vi "五子棋.vi"() -> ()   [LabVIEW 2018]
panel:
  in  "开始游戏":bool
  in  "对弈模式":enum16{"人机对弈", "双人对弈"}(ring)
  in  "重新开始":bool
  in  "退出程序":bool
  out "消息显示":string(combo)
  in  "控制数组":bool[][](array[boolean])
  out "显示数组":bool[][](array[boolean])
  out "当前棋盘状态":u16[][](array[ring])
  # "五  子  棋"
  # "0"
  # "1"
  # "2"
  # "3"
  # "4"
  # "5"
  # "6"
  # "7"
  # "8"
  # "9"
  # "10"
  # "11"
  # "12"
  # "13"
  # "14"
  # "0"
  # "1"
  # "2"
  # "3"
  # "4"
  # "5"
  # "6"
  # "7"
  # "8"
  # "9"
  # "10"
  # "11"
  # "12"
  # "13"
  # "14"
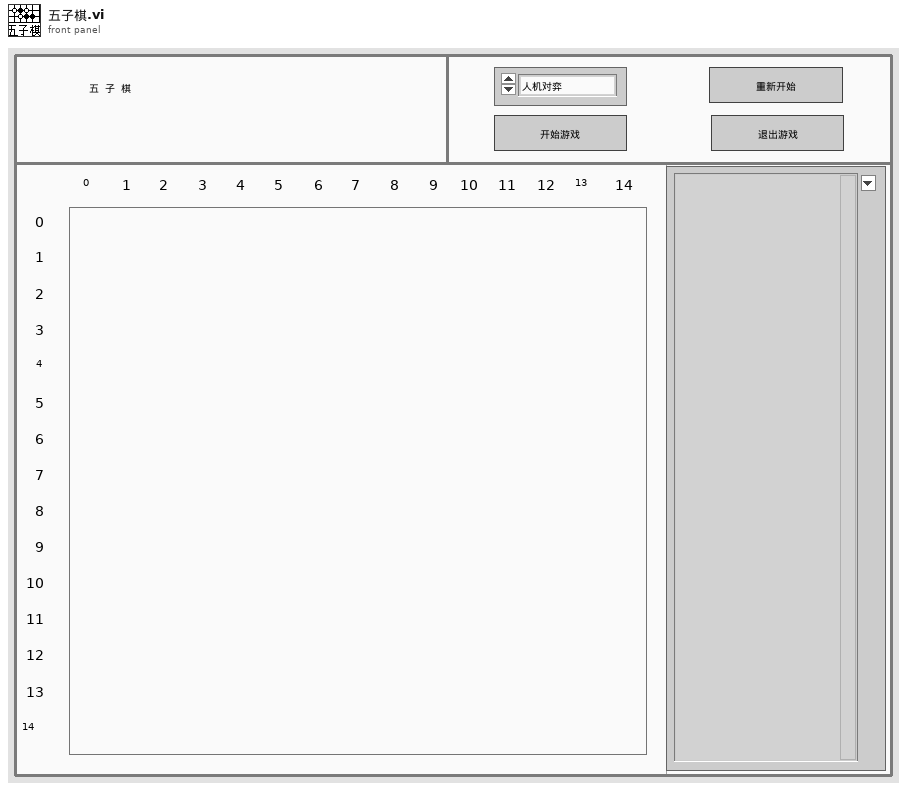
[diagram p1: front panel]
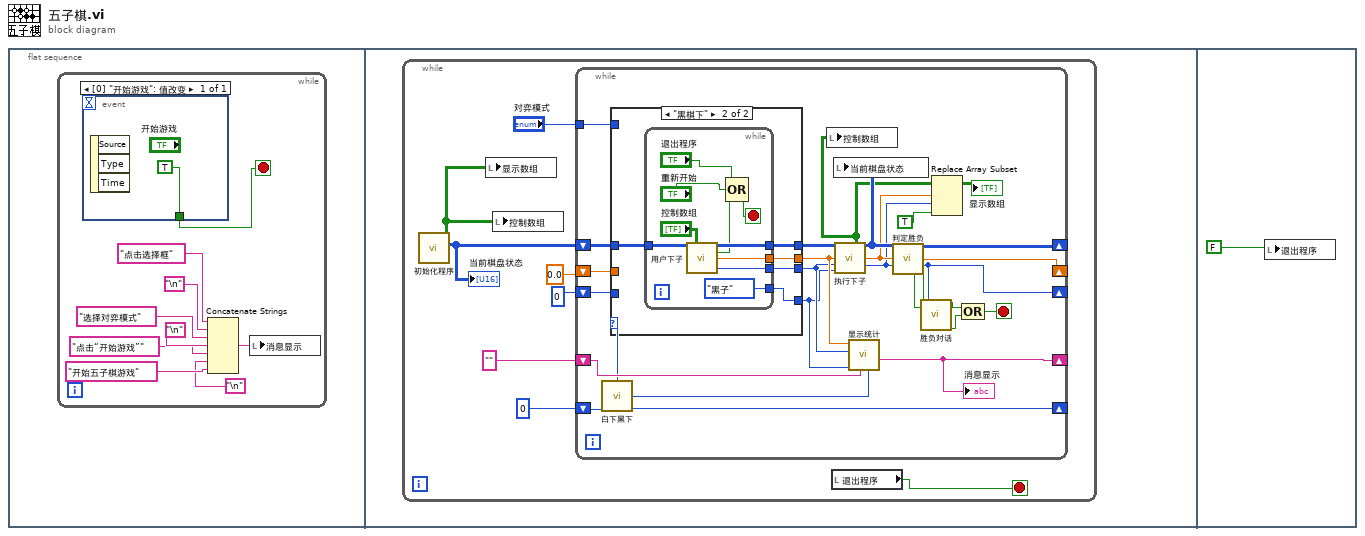
[diagram p0: block diagram]
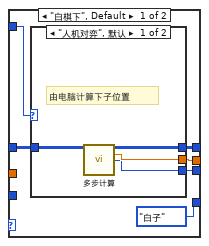
[diagram p2: hidden frame]
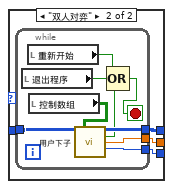
[diagram p3: hidden frame]
diagram:
  n1 = flat-sequence {
    frame #0 {
      n2 = while {
        stop <- w9 stop-if-true
        n3 = event shown="[0] \"开始游戏\": 值改变" {
          selector: _ -> [_]
          dyn-events: _ -> [_]
          timeout: _ -> [_]
          tunnel: [TRUE] -> w9
          event "开始游戏": Value Change {
            n4 = event-data() -> ()  [unwired: 1 in, 3 out]
          }
        }
        n5 = Concatenate Strings("点击选择框", "\n", "选择对弈模式", "\n", "点击“开始游戏”", "\n", "开始五子棋游戏") -> (w5:string)
        n6 = local write "消息显示"(w5) -> ()
      }
    }
    frame #1 {
      n7 = while {
        stop <- w13 stop-if-true
        n8 = call "初始化程序.vi"() -> ("当前棋盘状态"=w15:i32[][], "控制数组"=w14:bool[][])  [unwired: 1 in, 9 out]
        "当前棋盘状态" <- w15
        n9 = local write "显示数组"(w14) -> ()
        n10 = local write "控制数组"(w14) -> ()
        n11 = while {
          shift-right: [w39] -> _
          shift-left: 0 -> [w40]
          shift-right: [w41] -> _
          shift-left: sgl 0.0 -> [w46]
          shift-right: [w37] -> _
          shift-left: 0 -> [w45]
          shift-right: [w42] -> _
          shift-left: w15 -> [w44]
          shift-right: [w19] -> _
          shift-left: "" -> [w38]
          tunnel: "对弈模式" -> [w36]
          stop <- w43 stop-if-true
          n12 = call "白下黑下.vi"("下棋步数"=w40) -> ("Enum"=w24:enum16{"黑棋下", "白棋下"}, "下棋步数"=w23:i32, "黑白棋一共的下棋步数"=w39:i32)  [unwired: 2 in, 10 out]
          n13 = case shown="\"黑棋下\"" w24 {
            tunnel: [w50 w74] -> w35
            tunnel: [w49 w73] -> w33
            tunnel: [w48 w72] -> w32
            tunnel: [enum16{"白子", "无子", "黑子"}."白子" w71] -> w31
            tunnel: w46 -> [_ _]
            tunnel: w45 -> [_ _]
            tunnel: w44 -> [w51 w70]
            tunnel: w36 -> [w47 _]
            frame "白棋下", Default {
              n14 = case shown="\"人机对弈\", 默认" w47 {
                tunnel: w51 -> [w56 w60]
                tunnel: [w55 w59] -> w50
                tunnel: [w54 w58] -> w49
                tunnel: [w53 w57] -> w48
                frame "人机对弈", Default {
                  # "由电脑计算下子位置"
                  n15 = call "多步计算.vi"("输入棋盘状态"=w56) -> ("输出棋盘状态"=w55:i32[][], "最佳的行"=w54:sgl, "最佳的列"=w53:i16)  [unwired: 12 out]
                }
                frame "双人对弈" {
                  n16 = while {
                    tunnel: w60 -> [w69]
                    tunnel: [w68] -> w59
                    tunnel: [w67] -> w58
                    tunnel: [w66] -> w57
                    stop <- w64 stop-if-true
                    n17 = local read "退出程序"() -> (w62:bool)
                    n18 = local read "重新开始"() -> (w61:bool)
                    n19 = local read "控制数组"() -> (w63:bool[][])
                    n20 = call "用户下子.vi"("当前棋盘状态"=w69, "控制数组"=w63) -> ("当前棋盘状态"=w68:i32[][], "当前点可下?"=w65:bool, "行"=w67:sgl, "列"=w66:i16)  [unwired: 1 in, 9 out]
                    n21 = Compound Arithmetic op=OR(w61, w62, w65) -> (w64:bool)
                  }
                }
              }
            }
            frame "黑棋下" {
              n22 = while {
                tunnel: [w84] -> w74
                tunnel: [w83] -> w73
                tunnel: [w82] -> w72
                tunnel: [enum16{"白子", "无子", "黑子"}."黑子"] -> w71
                tunnel: w70 -> [w78]
                stop <- w79 stop-if-true
                n23 = call "用户下子.vi"("当前棋盘状态"=w78, "控制数组"="控制数组") -> ("当前棋盘状态"=w84:i32[][], "当前点可下?"=w80:bool, "行"=w83:sgl, "列"=w82:i16)  [unwired: 1 in, 9 out]
                n24 = Compound Arithmetic op=OR("退出程序", "重新开始", w80) -> (w79:bool)
              }
            }
          }
          n25 = call "执行下子.vi"("当前棋盘状态"=w35, "行"=w33, "列"=w32, "白子/黑子?"=w31) -> ("控制数组"=w30:bool[][], "当前棋盘状态"=w34:i32[][], "行"=w29:sgl, "列"=w28:i16)  [unwired: 8 out]
          n26 = local write "控制数组"(w30) -> ()
          n27 = local write "当前棋盘状态"(w34) -> ()
          n28 = call "显示统计.vi"("下棋步数"=w23, "前面下棋位置"=w38, "下子方？"=w31, "列"=w32, "行"=w33) -> ("下棋位置"=w19:string)  [unwired: 1 in, 5 out]
          "消息显示" <- w19
          n29 = call "判定胜负.vi"("当前棋盘状态"=w34, "行"=w29, "列"=w28) -> ("当前棋盘状态"=w42:i32[][], "行"=w41:sgl, "列"=w37:i16, "白子胜?"=w25:bool, "黑子胜?"=w26:bool)  [unwired: 8 out]
          n30 = call "胜负对话.vi"("黑子胜？"=w26, "白子胜？"=w25, "行或列"=w37) -> ("x .or. y?"=w21:bool, "退出循环？"=w20:bool)  [unwired: 15 out]
          n31 = Replace Array Subset(array=w30, new element=TRUE ("new element/subarray"), index (row)=w29, index (col)=w28) -> (→"显示数组":bool[][])
          n32 = Compound Arithmetic op=OR(w21, w20) -> (w43:bool)
        }
        n33 = local read "退出程序"() -> (w13:bool)
      }
    }
    frame #2 {
      n34 = local write "退出程序"(FALSE ("退出")) -> ()
    }
  }
